vi "Send Action to Core.vi"(8 "error in (no error)":errorcluster, 10 "AnyEvents":refnum<class "EventsAbstract.lvclass">, 11 "LogsAbstract in":refnum<class "LogsAbstract.lvclass">) -> (0 "error out":errorcluster, 3 "LogsAbstract out":refnum<class "LogsAbstract.lvclass">)   [LabVIEW 2019, in "LogsAbstract.lvlib" / "LogsAbstract.lvclass"]
uses:
  LogsAbstract.lvclass
  Classes/EventsAbstract/EventsAbstract.lvclass
  Modules/Core Messages/Action Handler Msg/Action Handler Msg.lvclass
  Modules/ModuleAbstract/ModuleAbstract.lvclass
  C:/Projekty/_Wewnetrzne/PC_ActorFramework/07_Program/LABVIEW/02_Source/Modules/ModuleAbstract/ModuleAbstract.lvclass
  C:/Program Files (x86)/National Instruments/LabVIEW 2019/vi.lib/MGI/Monitored Actor/Monitored Actor/Monitored Actor/Monitored Actor.lvclass
  C:/Program Files (x86)/National Instruments/LabVIEW 2019/vi.lib/ActorFramework/Actor/Actor.lvclass
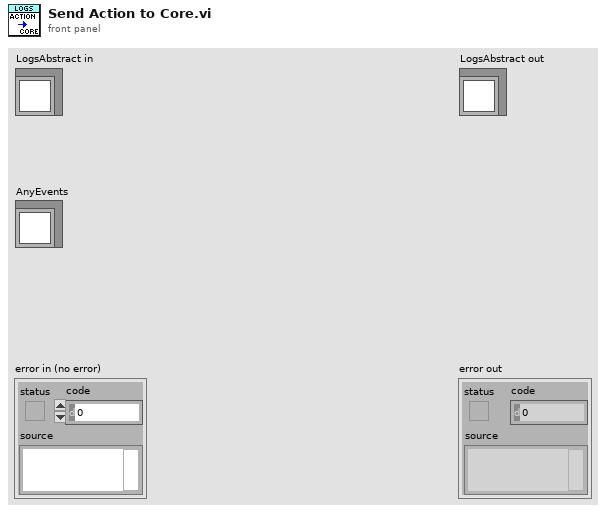
[diagram p1: front panel]
types:
  T1 = typedef "EventsAbstract.lvclass/Event Actions.ctl" = cluster{"Send Action":bool, "Broadcast Action":bool, "Action":T2, "Modules":cluster{"ModuleRef":refnum<class "Message Enqueuer.lvclass">, "UIRef":refnum<class "Message Enqueuer.lvclass">}[]}
  T2 = typedef "ModuleAbstract.lvlib/ModuleAbstract.lvclass/Module Actions.ctl" = enum16{"To Safe State", "Reset Safe State", "Close Module", "Close App"}
  T3 = cluster{"ModRef":refnum<class "Message Enqueuer.lvclass">, "UIRef":refnum<class "Message Enqueuer.lvclass">}
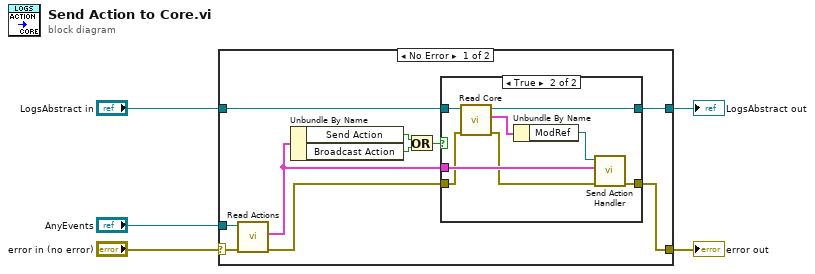
[diagram p0: block diagram]
diagram:
  n1 = case shown="No Error" "error in (no error)" {
    selector: "error in (no error)" -> [w14 w27]
    tunnel: [w6 w27] -> w4
    tunnel: [w10 w26] -> w2
    tunnel: "LogsAbstract in" -> [w9 w26]
    tunnel: "AnyEvents" -> [w15 _]
    frame No Error {
      n2 = call "Read Actions.vi"("error in (no error)"=w14, "EventsAbstract in"=w15) -> ("error out"=w7:errorcluster, "Actions"=w8:T1)  [unwired: 7 in, 1 out]
      n3 = Unbundle By Name(w8) -> ("Send Action"=w12:bool, "Broadcast Action"=w13:bool)
      n4 = Or(x=w12, y=w13) -> (x .or. y?=w11:bool)
      n5 = case shown="True" w11 {
        tunnel: [w17 w23] -> w10
        tunnel: w9 -> [w17 w22]
        tunnel: w8 -> [_ w25]
        tunnel: w7 -> [w16 w19]
        tunnel: [w16 w24] -> w6
        frame False {
        }
        frame True {
          n6 = call "Read Core.vi"("error in (no error)"=w19, "ModuleAbstract in"=w22) -> ("error out"=w18:errorcluster, "Core"=w21:T3, "ModuleAbstract out"=w23:refnum<class "LogsAbstract.lvclass">)  [unwired: 7 in]
          n7 = Unbundle By Name(w21) -> ("ModRef"=w20:refnum<class "Message Enqueuer.lvclass">)
          n8 = call "Send Action Handler.vi"("error in (no error)"=w18, "Actions"=w25, "Message Enqueuer"=w20) -> ("error out"=w24:errorcluster)  [unwired: 7 in, 1 out]
        }
      }
    }
    frame Error {
    }
  }
  "error out" <- w4
  "LogsAbstract out" <- w2
